vi "_Serial_Mark10-Setup(Zero).vi"(5 "Serial Port":refnum<visa-resource-name>="COM5") -> (2 "VISA resource name out":refnum<visa-resource-name>)   [LabVIEW 2015]
panel:
  out "에러 출력":errorcluster
  out "TX String":string
  # "MARK10 moving speed control"
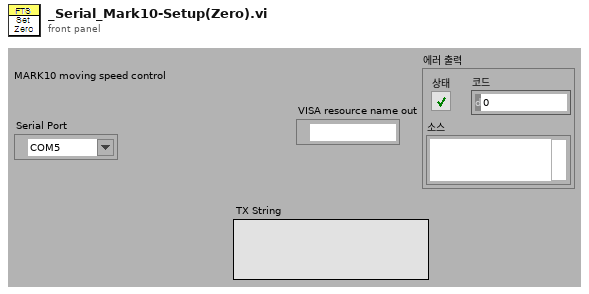
[diagram p1: front panel]
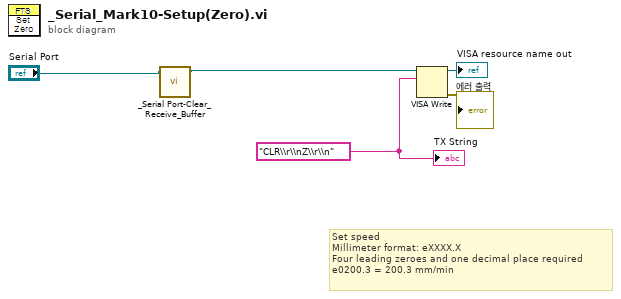
[diagram p0: block diagram]
diagram:
  w2 = "CLR\\r\\nZ\\r\\n" ("포맷 문자열")
  # "Set speed\nMillimeter format: eXXXX.X\nFour leading zeroes and one decimal place required\ne0200.3 = 200.3 mm/min"
  n1 = call "_Serial Port-Clear_Receive_Buffer.vi"("Serial Port"="Serial Port") -> ("Serial Port out"=w3:refnum<visa-resource-name>)  [unwired: 3 in, 1 out]
  n2 = VISA Write(VISA resource name=w3, write buffer=w2) -> (VISA resource name out=→"VISA resource name out":refnum<visa-resource-name>, error out=→"에러 출력":errorcluster)  [unwired: 1 in, 1 out]
  "TX String" <- w2
